vi "Test cwDrift.vi"() -> ()   [LabVIEW 2020]
uses:
  Labview Library/Libraries/Basic Experiment/CW settings.ctl
  Labview Library/Libraries/Read TDMS Data/Library/Write CSV Property_Path.vi
  Labview Library/Libraries/Read TDMS Data/Library/Write CSV Property_Numeric.vi
  <vilib>/Utility/file.llb/Write Delimited Spreadsheet (string).vi
  Labview Library/Libraries/Basic Experiment/Basic Experiment.lvlib
  Labview Library/Libraries/Read TDMS Data/Library/Read TDMS Data.lvlib
panel:
  in  "Result Path":path=path "G:/Exp_Log/2023_12_03_Align_Magnetic_Field_AlongVV/SN23_07_27_ 806_CWdrift.csv"
  in  "Settings":T1={"Num Pts"=20, "Start freq"=1099.0, "Stop freq"=1111.0, " dBm"=-5.0, "Ratio \nThre(abs)"=0.03, "AutoTrace Before Exp"=TRUE, "RepoSave"=FALSE, "Peak Num \nLimit "=1, "Loop per Update"=1200, "UpdateTime"=80} {"UpdateTime" format="%.0p"; "Loop per Update" format="%#_6p"}
  in  "stop":bool
  # "CW Settings"
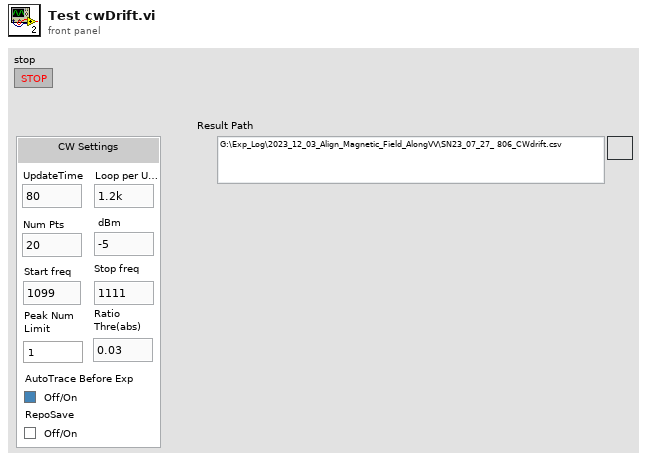
[diagram p1: front panel]
types:
  T1 = typedef "Basic Experiment.lvlib/CW settings.ctl" = cluster{"Num Pts":i32, "Start freq":dbl, "Stop freq":dbl, " dBm":dbl, "Ratio \nThre(abs)":dbl, "AutoTrace Before Exp":bool, "RepoSave":bool, "Peak Num \nLimit ":i32, "Loop per Update":u32, "UpdateTime":i32}
  T2 = typedef "Basic Experiment.lvlib/CW Results.ctl" = cluster{"Fit Frequency":T3, "Pro":dbl[], "Error Bar":dbl[], "Raw Data Path":path, "Image Path":path}
  T3 = typedef "Basic Experiment.lvlib/CW Fit Frequency.ctl" = cluster{"Fre2":cluster{"Amplitude":dbl, "Position":dbl, "Width":dbl}, "Fre1":cluster{"Amplitude":dbl, "Position":dbl, "Width":dbl}, "Fre3":cluster{"Amplitude":dbl, "Position":dbl, "Width":dbl}, "Background":dbl}
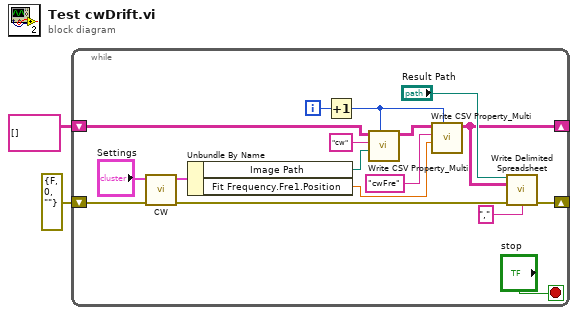
[diagram p0: block diagram]
diagram:
  n1 = while {
    shift-right: [w9] -> _
    shift-left: errorcluster {"status"=FALSE, "code"=0, "source"=""} ("error out") -> [w17]
    shift-right: [w6] -> _
    shift-left: string[][] [] ("Csv output") -> [w8]
    i -> [w16]
    stop <- "stop" stop-if-true
    n2 = call "CW.vi"("error in (no error)"=w17, "Settings"="Settings") -> ("error out"=w10:errorcluster, "CW Result"=w15:T2)  [unwired: 7 in, 1 out]
    n3 = Unbundle By Name(w15) -> ("Image Path"=w14:path, "Fit Frequency.Fre1.Position"=w4:dbl)
    n4 = Increment(x=w16) -> (x+1=w5:i32)
    n5 = call-poly "Write CSV Property_Multi.vi"("Index(NewLine)"=w5, "File Path"=w14, "Property Name"="cw", "Csv input"=w8) -> ("Csv output"=w7:string[][])  [unwired: 7 in]
    n6 = call-poly "Write CSV Property_Multi.vi"("Index(NewLine)"=w5, "Property Value"=w4, "Property Name"="cwFre", "Csv input"=w7) -> ("Csv output"=w6:string[][])  [unwired: 7 in]
    n7 = call-poly <vilib>:"Write Delimited Spreadsheet.vi"("file path (dialog if empty)"="Result Path", "2D data"=w6, "error in (no error)"=w10, "delimiter (\\t)"="," ("delimiter (\\t)")) -> ("error out"=w9:errorcluster)  [unwired: 10 in, 1 out]
  }
